vi "ATA_RT_2017_07_28.vi"() -> ()   [LabVIEW 2018]
doc: "This VI transfers a finite number of samples from the FPGA target to the Host using a stream."
uses:
  <vilib>/rvi/interface/nirviMethod/nirviMethod.xnode
  <vilib>/rvi/interface/nirviOpenFPGA/nirviOpenFPGA.xnode
  <vilib>/rvi/interface/nirviCloseFPGA/nirviCloseFPGA.xnode
  <vilib>/rvi/errors/niLvFpgaMergeErrorWithErrorCode.vi
  <vilib>/rvi/interface/nirviReadWriteControl/nirviReadWriteControl.xnode
  <vilib>/Analysis/NI_AALPro.lvlib
  <vilib>/FPGAPlugInAG/Dynamic/niLvFpga_ReadFifo_Dynamic.vi
  <vilib>/rvi/Analysis/host/Public/NI_FpgaMspHost.lvlib
  <vilib>/Analysis/2dsp.llb/Real FFT.vi
  <vilib>/FPGAPlugInAG/Dynamic/niLvFpga_StartFifo_Dynamic.vi
  <vilib>/rvi/interface/Simulation/niFpgaSimulationCallBeginRW.vi
  <vilib>/rvi/errors/niLvFpgaAdjustHostInterfaceError.vi
  ProjectFiles/FPGA Bitfiles/20170803_00_ATA_FPGA_00.lvbitx
  <vilib>/FPGAPlugInAG/Dynamic/niLvFpga_ConfigureFifo_Dynamic.vi
  NiFpgaLv.dll
  <vilib>/FPGAPlugInAG/Dynamic/niLvFpga_Close_Dynamic.vi
  Controls/DataClass.ctl
  <vilib>/Analysis/4window.llb/Hanning Window (DBL).vi
  Controls/ToneInfoClust.ctl
  <vilib>/FPGAPlugInAG/PXIe-7976R/niLvFpga_Open_PXIe-7976R.vi
  <vilib>/rvi/interface/common/dynamic/niFpgaDynamicAddResources.vi
panel:
  out "concatenated string":string
  out "FreqShiftTab":enum32{"Auto", "Manual"}(tab)=enum."Manual"
  in  "CoarseShift":dbl(slide)=-24999000.0 caption="Frequency Shift Coarse (Hz)" scale=-26000000.0..-23000000.0 scale format="%^#_6g"
  in  "FineShift":dbl(slide)=-462.63345195729516 caption="Frequency Shift Fine (Hz)" scale=-10000.0..10000.0 scale format="%^#_6g"
  in  "ProbesTab":T1(tab)=enum."Enable Stages"
  in  "EnableStep1":bool=TRUE
  in  "ScaleMeasurement":fxp<+/-,23,23>=10000.0
  in  "Scale_In_RT":ext=1.0
  in  "Scale_Step1":fxp<+/-,23,23>=4194303.0
  in  "Scale_NoiseFloor":fxp<+/-,23,23>=4194303.0
  in  "Offset":fxp<+/-,16,1>=0.000213623046875
  in  "FlushQ":bool=TRUE
  in  "Enable":T2={"FreqShiftEnable"=TRUE, "Step4Enable"=TRUE, "Step5Enable"=TRUE, "Step6Enable"=TRUE, "Step7Enable"=TRUE}
  in  "Scale":T3={"Scale_Step4"=10.0, "Scale_Step5"=1.0, "Scale_Step6"=1.0, "Scale_Step7"=1.0}
  out "Probe 1":i16=-13
  out "Probe 2":fxp<+/-,16,1>=-0.000274658203125
  out "Probe 3":fxp<+/-,39,24>=1.52587890625
  out "Probe 4":fxp<+/-,16,1>
  out "Probe 5":fxp<+/-,40,2>=-0.004281044006347656
  out "Probe 6":fxp<+/-,63,25>=9180.997811079025
  out "Probe 7":fxp<+/-,63,1>=6.103514169808477e-05
  out "Probe 21":fxp<+/-,24,3>=0.008556365966796875 format="%.2p"
  out "Probe 22":fxp<+/-,47,26>=4411.998948097229
  out "Probe 23":fxp<+/-,47,1>=-0.0003757475910788344
  out "Probe 24":fxp<+/-,16,1>=0.000213623046875
  out "Probe":T4={"Probe 8"=0.00049591064453125, "Probe 9"=0.0051984291058033705, "Probe 10"=0.051984291058033705, "Probe 11"=0.023252144874277292, "Probe 12"=0.023252144874277292, "Probe 13"=0.023252144874277292, "Probe 14"=0.015486729560507229, "Probe 15"=0.015486729560507229, "Probe 16"=0.015486729560507229, "Probe 17"=0.003276327208368457, "Probe 18"=0.003276327208368457, "Probe 19"=0.003276327208368457, "Probe20"=0.003276327208368457}
  out "TransferCount":u64=226407353343
  out "#Transfers":i32=74
  out "#FFTs":i32=74
  out "Elements Remaining":u32
  out "Peak Location":dbl=25000106.633451957 format="%^#_11g"
  out "SampleRate":dbl=12500.0
  out "max value":dbl=4.648353358875404e-06
  out "max index(es)":i32=644
  out "FAM Initialized?":bool=TRUE
  out "Total Shift":dbl=-24999462.633451957
  in  "AutoCenter":bool
  in  "Tab Control 2":T5(tab)
  out "NoiseFloor 2":ext[](graph)
  out "NoiseFloor":dbl[](graph)
  out "df (Hz) 2":dbl=7629.39453125
  out "NoiseFloorLoopCount":i32=77
  in  "Noise Floor":u8(slide)=1 scale=0.0..1.0
  out "TimeDomain":ext[](graph)
  out "Filtered Spectrum":dbl[](graph)
  out "df (Hz)":dbl=1.0
  in  "Zoom On Peak":bool
  in  "Tones":u8(slide)=1 scale=0.0..1.0
  in  "stop":bool
  # "Log"
  # "Linear"
  # "Log"
  # "Linear"
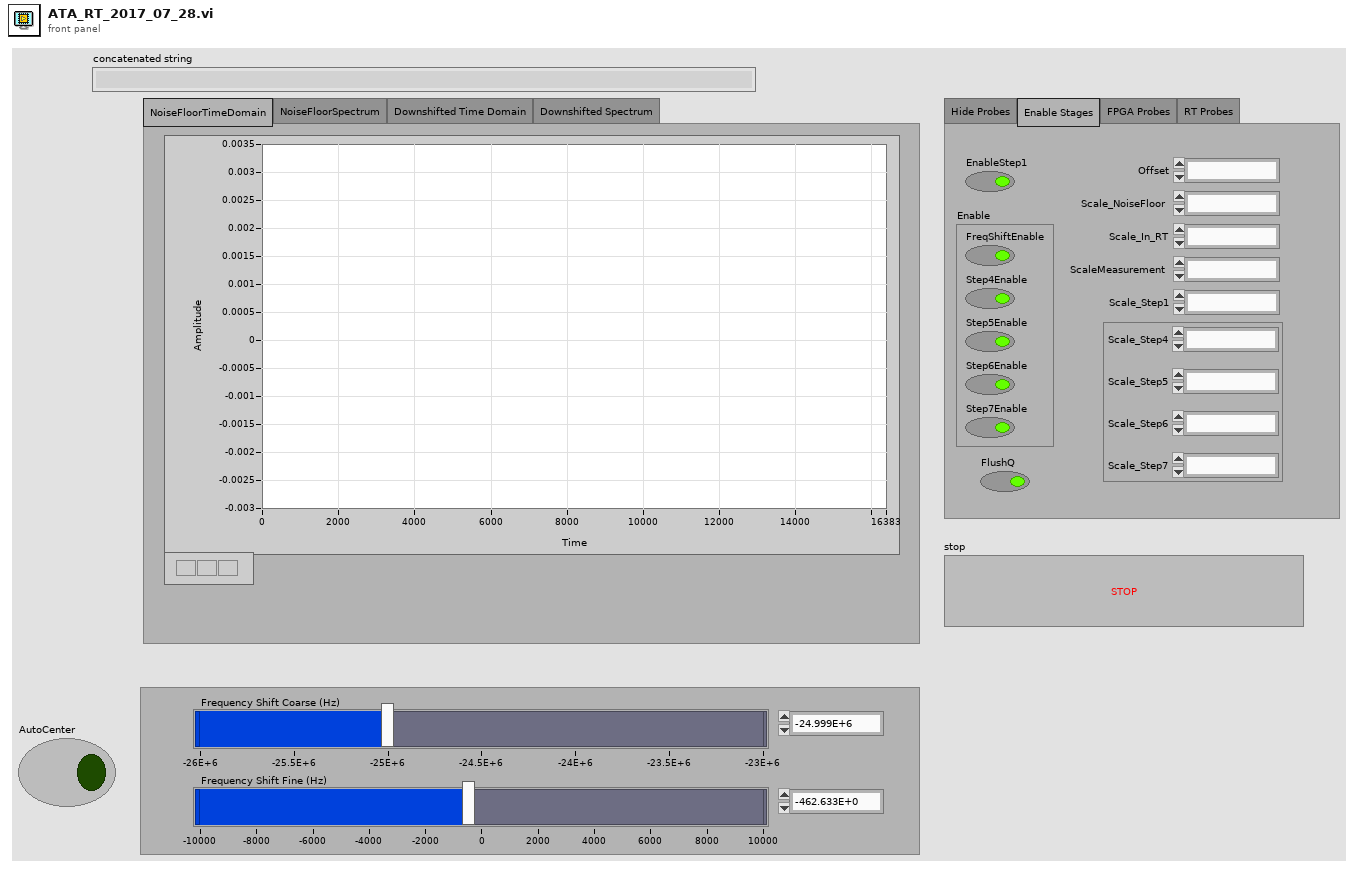
[diagram p1: front panel]
types:
  T1 = enum32{"Hide Probes", "Enable Stages", "FPGA Probes", "RT Probes"}
  T2 = cluster{"FreqShiftEnable":bool, "Step4Enable":bool, "Step5Enable":bool, "Step6Enable":bool, "Step7Enable":bool}
  T3 = cluster{"Scale_Step4":fxp<+/-,23,23>, "Scale_Step5":fxp<+/-,23,23>, "Scale_Step6":fxp<+/-,23,23>, "Scale_Step7":fxp<+/-,23,23>}
  T4 = cluster{"Probe 8":fxp<+/-,18,1>, "Probe 9":fxp<+/-,40,1>, "Probe 10":fxp<+/-,40,1>, "Probe 11":fxp<+/-,40,1>, "Probe 12":fxp<+/-,63,24>, "Probe 13":fxp<+/-,40,1>, "Probe 14":fxp<+/-,40,1>, "Probe 15":fxp<+/-,63,24>, "Probe 16":fxp<+/-,40,1>, "Probe 17":fxp<+/-,40,1>, "Probe 18":fxp<+/-,63,24>, "Probe 19":fxp<+/-,40,1>, "Probe20":fxp<+/-,40,1>}
  T5 = enum32{"NoiseFloorTimeDomain", "NoiseFloorSpectrum", "Downshifted Time Domain", "Downshifted Spectrum"}
  T6 = enum16{"open", "replace", "create", "open or create", "replace or create", "replace or create with confirmation"}
  T7 = typedef "DataClass.ctl" = enum16{"Tone", "Noise"}
  T8 = typedef "ToneInfoClust.ctl" = cluster{"PkLocTrak":dbl, "PkLocDisp":dbl, "df_":dbl, "ZoomPwr":dbl[], "Phase":dbl, "PhaseOld":dbl, "AboveThresh?":bool, "MaxI":dbl, "MaxQ":dbl, "median":dbl, "ISpect":dbl[], "QSpect":dbl[], "DeltaPhase":dbl}
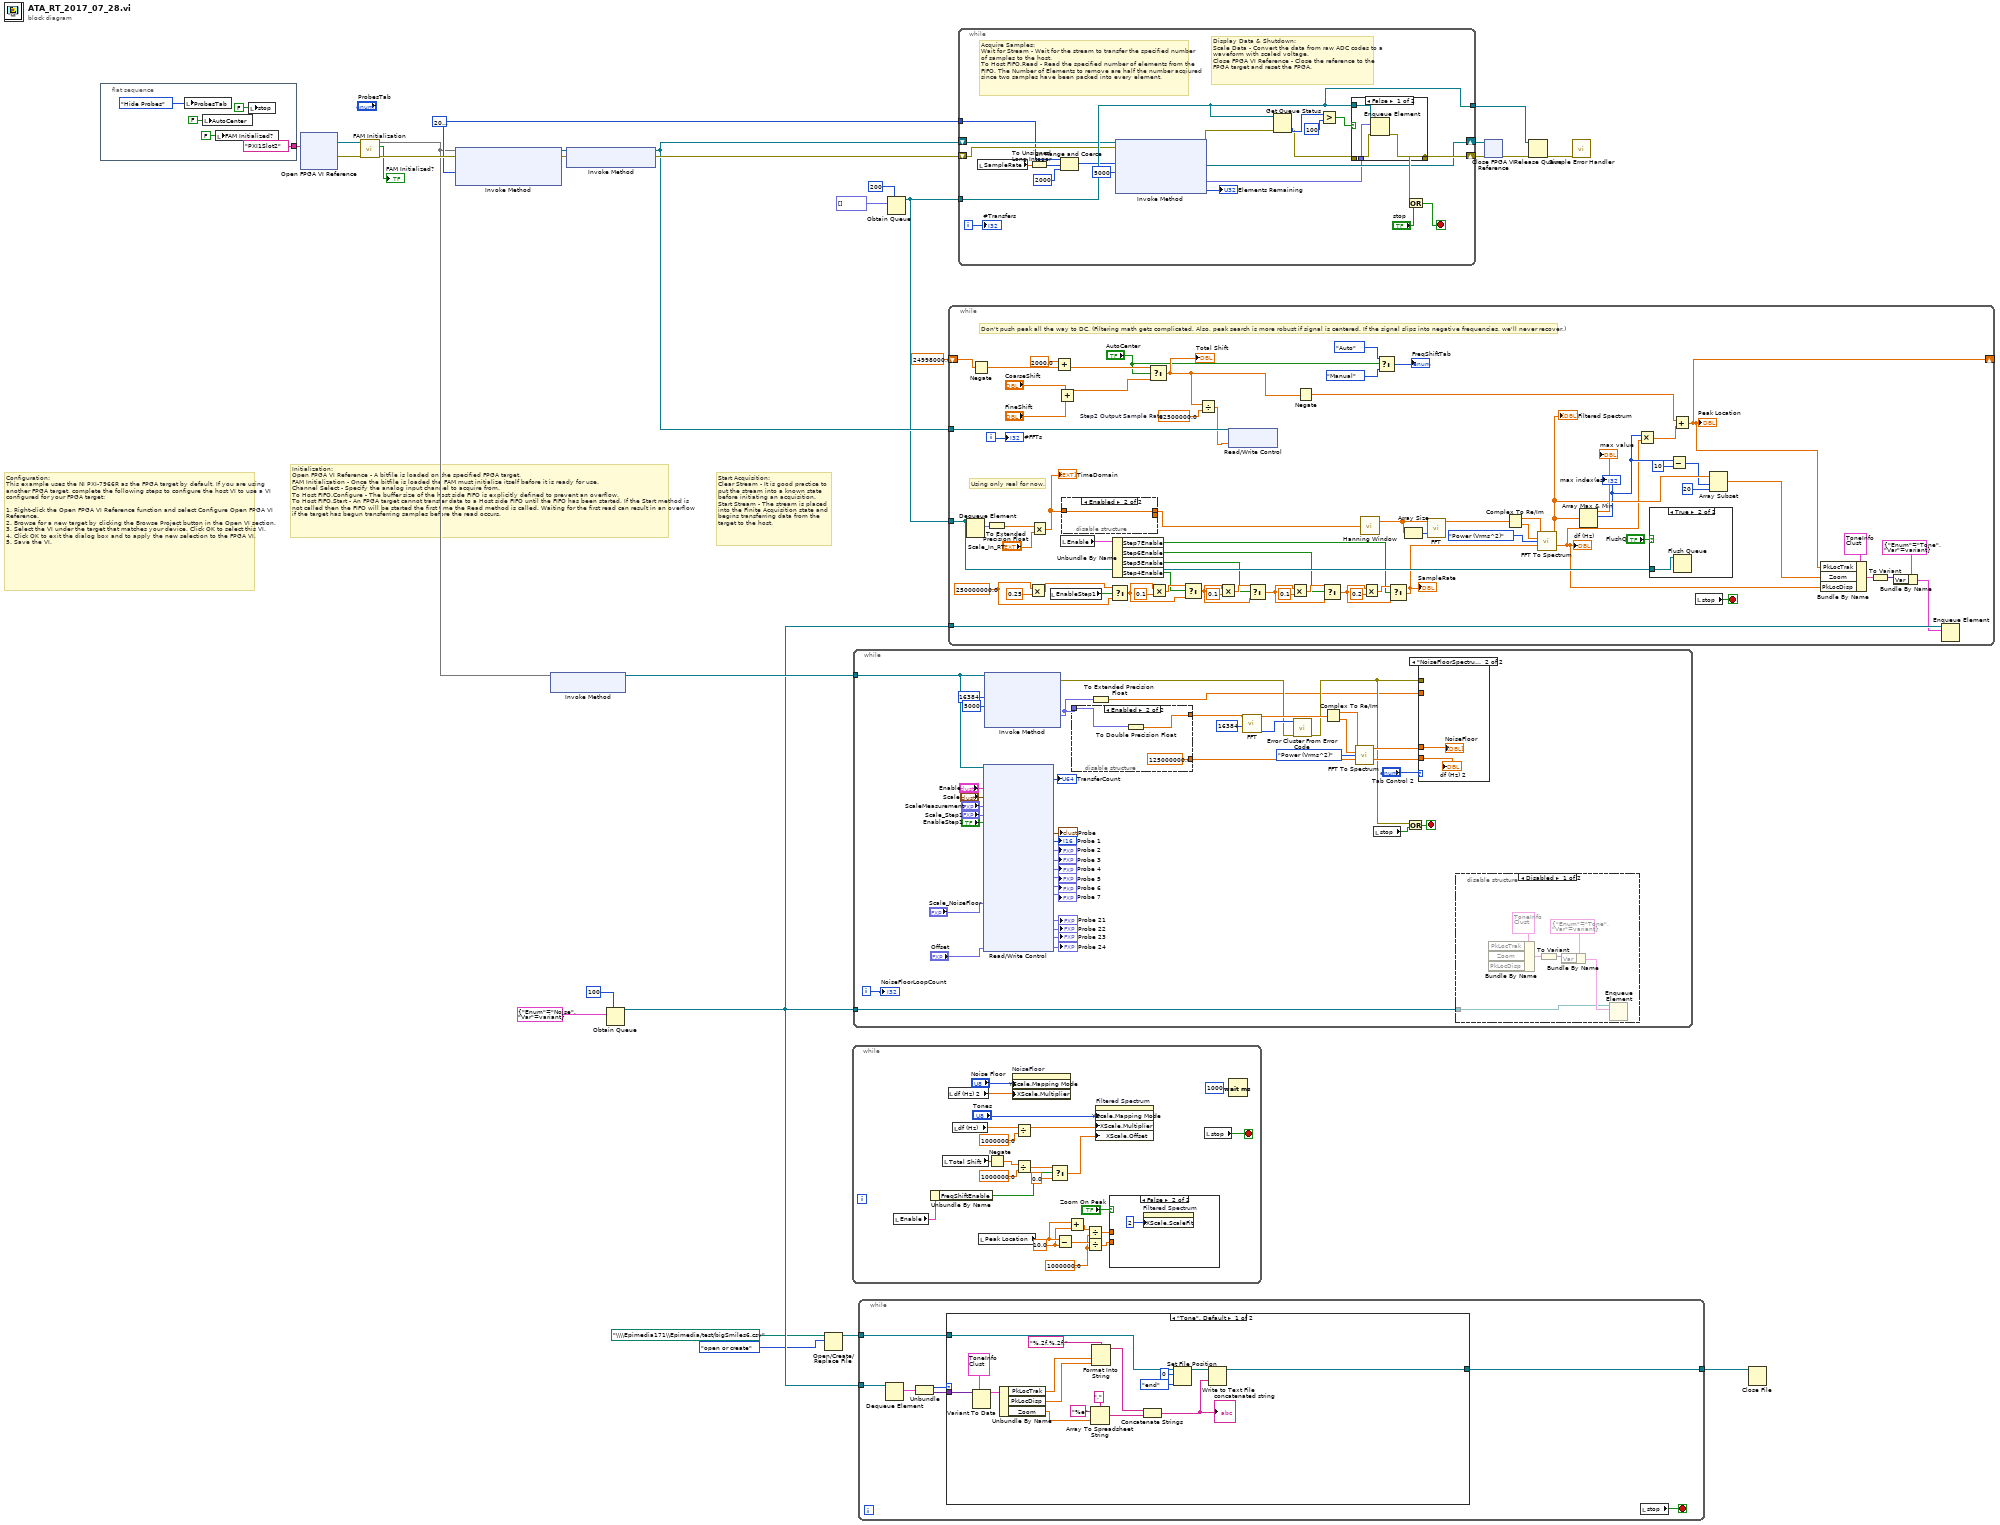
[diagram p0: block diagram]
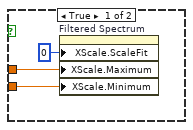
[diagram p3: hidden frame]
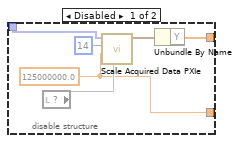
[diagram p5: hidden frame]
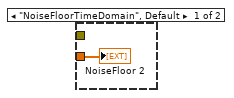
[diagram p6: hidden frame]
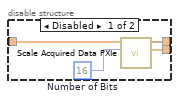
[diagram p7: hidden frame]
diagram:
  w18 = u32 2000000 ("Num Samples")
  # "Start Acquisition:\nClear Stream - It is good practice to put the stream into a known state before initiating an acquisition.\nStart Stream - The stream is placed into the Finite Acquisition state and begins transferring data from the target to the host."
  # "Initialization:\nOpen FPGA VI Reference - A bitfile is loaded on the specified FPGA target.\nFAM Initialization - Once the bitfile is loaded the FAM must initialize itself before it is ready for use.\nChannel Select - Specify the analog input channel to acquire from.\nTo Host FIFO.Configure - The buffer size of the host side FIFO is explicitly defined to prevent an overflow.\nTo Host FIFO.Start - An FPGA target cannot transfer data to a Host side FIFO until the FIFO has been started. If the Start method is not called then the FIFO will be started the first time the Read method is called. Waiting for the first read can result in an overflow if the target has begun transferring samples before the read occurs."
  # "Configuration:\nThis example uses the NI PXI-7966R as the FPGA target by default. If you are using another FPGA target, complete the following steps to configure the host VI to use a VI configured for your FPGA target:\n\n1. Right-click the Open FPGA VI Reference function and select Configure Open FPGA VI Reference.\n2. Browse for a new target by clicking the Browse Project button in the Open VI section.\n3. Select the VI under the target that matches your device. Click OK to select this VI.\n4. Click OK to exit the dialog box and to apply the new selection to the FPGA VI.\n5. Save the VI."
  n1 = flat-sequence {
    tunnel: [tag "PXI1Slot2" ("resource name")] -> w9
    frame #0 {
      n2 = local write "ProbesTab"(T1."Hide Probes" ("ProbesTab")) -> ()
      n3 = local write "AutoCenter"(FALSE ("AutoCenter")) -> ()
      n4 = local write "FAM Initialized?"(FALSE ("FAM Initialized?")) -> ()
      n5 = local write "stop"(FALSE ("stop")) -> ()
    }
  }
  n6 = xnode ("Open FPGA VI Reference")("resource name"=w9) -> ("FPGA VI Reference Out"=w19:refnum<k20>, "error out"=w24:errorcluster)  [unwired: 1 in]
  n7 = call "FAM Initialization.vi"("error in (no error)"=w24, "Cluster"=w19) -> ("error out"=w28:errorcluster, "FAM Initialized?"=→"FAM Initialized?":bool, 3:w11)  [unwired: 7 in]
  n8 = xnode "Invoke Method"("FPGA VI Reference In"=w11, "error in"=w28, "Requested Depth"=w18) -> ("FPGA VI Reference Out"=w26:refnum<k20>, "error out"=w25:errorcluster)  [unwired: 1 out]
  n9 = xnode "Invoke Method"("FPGA VI Reference In"=w11) -> ("FPGA VI Reference Out"=w10:refnum<k20>)  [unwired: 1 in, 1 out]
  n10 = xnode "Invoke Method"("FPGA VI Reference In"=w26, "error in"=w25) -> ("FPGA VI Reference Out"=w22:refnum<k20>, "error out"=w23:errorcluster)
  n11 = Obtain Queue(max queue size (-1, unlimited)=100, element data type=cluster{"Enum":T7, "Var":variant} {"Enum"=enum."Noise", "Var"=variant}) -> (queue out=w5:refnum<queue>)  [unwired: 3 in, 2 out]
  n12 = Open/Create/Replace File(file path (use dialog)=path "\\\\Epimedia171\\Epimedia/test/bigSmiles6.csv" ("file (use dialog)"), operation (0:open)=T6."open or create") -> (refnum out=w3:refnum<file>)  [unwired: 4 in, 2 out]
  n13 = while {
    stop <- w57 stop-if-true
    w39 = 1000000.0 ("x")
    w45 = 10.0 ("y")
    n14 = local read "Enable"() -> (w36:T2)
    n15 = Unbundle By Name(w36) -> ("FreqShiftEnable"=w35:bool)
    n16 = local read "Total Shift"() -> (w51:dbl)
    n17 = local read "df (Hz) 2"() -> (w52:dbl)
    n18 = local read "df (Hz)"() -> (w53:dbl)
    n19 = local read "Peak Location"() -> (w46:dbl)
    n20 = Negate(x=w51) -> (-x=w48:dbl)
    n21 = property on="NoiseFloor" class="WFGraph (strict)"("YScale.Mapping Mode"="Noise Floor", "XScale.Multiplier"=w52) -> ()  [unwired: 2 in, 2 out]
    n22 = Divide(x=w53, y=1000000.0) -> (x/y=w50:dbl)
    n23 = Divide(x=w48, y=1000000.0) -> (x/y=w38:dbl)
    n24 = Select(t=w38, s=w35, f=0.0) -> (s? t:f=w37:dbl)
    n25 = Subtract(x=w46, y=w45) -> (x-y=w41:dbl)
    n26 = Add(x=w46, y=w45) -> (x+y=w44:dbl)
    n27 = Divide(x=w44, y=w39) -> (x/y=w42:dbl)
    n28 = Divide(x=w41, y=w39) -> (x/y=w40:dbl)
    n29 = property on="Filtered Spectrum" class="WFGraph (strict)"("YScale.Mapping Mode"="Tones", "XScale.Multiplier"=w50, "XScale.Offset"=w37) -> ()  [unwired: 2 in, 2 out]
    n30 = case shown="False" "Zoom On Peak" {
      tunnel: w40 -> [w60 _]
      tunnel: w42 -> [w59 _]
      frame True {
        n31 = property on="Filtered Spectrum" class="WFGraph (strict)"("XScale.ScaleFit"=u8 0 ("X Scale.Scale Fit"), "XScale.Maximum"=w59, "XScale.Minimum"=w60) -> ()  [unwired: 2 in, 2 out]
      }
      frame False {
        n32 = property on="Filtered Spectrum" class="WFGraph (strict)"("XScale.ScaleFit"=u8 2 ("X Scale.Scale Fit")) -> ()  [unwired: 2 in, 2 out]
      }
    }
    n33 = local read "stop"() -> (w57:bool)
    n34 = Wait (ms)(milliseconds to wait=u32 1000) -> ()  [unwired: 1 out]
  }
  n35 = while {
    tunnel: w10 -> [w86]
    tunnel: w5 -> [w62]
    i -> [w92]
    stop <- w90 stop-if-true
    n36 = xnode "Read/Write Control"("FPGA VI Reference In"=w86, "Enable"="Enable", "Scale"="Scale", "ScaleMeasurement"="ScaleMeasurement", "Scale_Step1"="Scale_Step1", "EnableStep1"="EnableStep1", "Scale_NoiseFloor"="Scale_NoiseFloor", "Offset"="Offset") -> ("TransferCount"=→"TransferCount":u64, "Probe"=→"Probe":T4, "Probe 1"=→"Probe 1":i16, "Probe 2"=→"Probe 2":fxp<+/-,16,1>, "Probe 3"=→"Probe 3":fxp<+/-,39,24>, "Probe 4"=→"Probe 4":fxp<+/-,16,1>, "Probe 5"=→"Probe 5":fxp<+/-,40,2>, "Probe 6"=→"Probe 6":fxp<+/-,63,25>, "Probe 7"=→"Probe 7":fxp<+/-,63,1>, "Probe 21"=→"Probe 21":fxp<+/-,24,3>, "Probe 22"=→"Probe 22":fxp<+/-,47,26>, "Probe 23"=→"Probe 23":fxp<+/-,47,1>, "Probe 24"=→"Probe 24":fxp<+/-,16,1>)  [unwired: 1 in, 2 out]
    n37 = xnode "Invoke Method"("FPGA VI Reference In"=w86, "Number of Elements"=u32 16384, "Timeout (ms)"=5000) -> ("error out"=w88:errorcluster, "Data"=w84:fxp<+/-,16,1>[])  [unwired: 1 in, 2 out]
    n38 = disable-structure shown="Enabled" {
      disable-tunnel: [w115 w118] -> w94
      disable-tunnel: w84 -> [w114 w119]
      disable-tunnel: [w112 125000000.0 ("sample rate (S/s)")] -> w81
      frame Disabled {
        w112 = 125000000.0
        n39 = local read item#-1() -> (w116)
        n40 = call "Scale Acquired Data PXIe.vi"("range (V)"=w116, "Sample Rate"=w112, "Number of Bits"=i16 14, "Data In"=w114) -> ("Data Out"=w113:waveform(dbl))  [unwired: 6 in, 1 out]
        n41 = Unbundle By Name(w113) -> ("Y"=w115:dbl[])
      }
      frame Enabled {
        n42 = To Double Precision Float(number=w119) -> (double precision float=w118:dbl[])
      }
    }
    n43 = To Extended Precision Float(1:w84) -> (0:w83:ext[])
    n44 = call-poly <vilib>:"FFT.vi"("FFT size"=16384, "X"=w94) -> ("error"=w89:i32, "FFT {X}"=w98:cdb[])  [unwired: 8 in]
    n45 = call <vilib>:"Error Cluster From Error Code.vi"("error in (no error)"=w88, "error code (0)"=w89) -> ("error out"=w87:errorcluster)  [unwired: 7 in]
    n46 = Complex To Re/Im(x + iy=w98) -> (x=w99:dbl[], y=w100:dbl[])
    n47 = call <vilib>:"FFT To Spectrum.vi"("real FFT data"=w99, "imaginary FFT data"=w100, "spectrum type"=enum8{"Power (Vrms^2)", "Amplitude (Vrms)"}."Power (Vrms^2)", "sample rate (S/s)"=w81) -> ("spectrum out"=w97:dbl[], "df (Hz)"=w96:dbl)  [unwired: 9 in, 1 out]
    n48 = local read "stop"() -> (w91:bool)
    n49 = Or(x=w87, y=w91) -> (x .or. y?=w90:bool)
    n50 = case shown="\"NoiseFloorSpectrum\"" "Tab Control 2" {
      tunnel: w97 -> [_ w122]
      tunnel: w96 -> [_ w121]
      tunnel: w83 -> [w120 _]
      tunnel: w87 -> [_ _]
      frame "NoiseFloorTimeDomain", Default {
        "NoiseFloor 2" <- w120
      }
      frame "NoiseFloorSpectrum" {
        "NoiseFloor" <- w122
        "df (Hz) 2" <- w121
      }
    }
    n51 = disable-structure shown="Disabled" {
      disable-tunnel: w62 -> [w104 _]
      frame Disabled {
        n52 = Bundle By Name(cluster=T8 {"PkLocTrak"=0.0, "PkLocDisp"=0.0, "df_"=0.0, "ZoomPwr"=[], "Phase"=0.0, "PhaseOld"=0.0, "AboveThresh?"=FALSE, "MaxI"=0.0, "MaxQ"=0.0, "median"=0.0, "ISpect"=[], "QSpect"=[], "DeltaPhase"=0.0}) -> (w109:T8, "PkLocTrak"=w106:dbl)  [unwired: 2 in]
        n53 = To Variant(anything=w109) -> (Variant=w108:variant)
        n54 = Bundle By Name(cluster=cluster{"Enum":T7, "Var":variant} {"Enum"=enum."Tone", "Var"=variant} ("element"), "Var"=w108) -> (w110:cluster{"Enum":T7, "Var":variant})
        n55 = Enqueue Element(queue=w104, element=w110) -> ()  [unwired: 2 in, 3 out]
      }
      frame Enabled {
      }
    }
    "NoiseFloorLoopCount" <- w92
  }
  n56 = while {
    tunnel: w5 -> [w128]
    tunnel: w3 -> [w124]
    tunnel: [w123] -> w2
    stop <- w129 stop-if-true
    n57 = Dequeue Element(queue=w128) -> (element=w127:cluster{"Enum":T7, "Var":variant})  [unwired: 2 in, 3 out]
    n58 = Unbundle(w127) -> ("Enum"=w126:T7, "Var"=w125:variant)
    n59 = case shown="\"Tone\", Default" w126 {
      tunnel: w125 -> [w146 _]
      tunnel: w124 -> [w141 w147]
      tunnel: [w137 w147] -> w123
      frame "Tone", Default {
        n60 = Variant To Data(type=T8 {"PkLocTrak"=0.0, "PkLocDisp"=0.0, "df_"=0.0, "ZoomPwr"=[], "Phase"=0.0, "PhaseOld"=0.0, "AboveThresh?"=FALSE, "MaxI"=0.0, "MaxQ"=0.0, "median"=0.0, "ISpect"=[], "QSpect"=[], "DeltaPhase"=0.0}, Variant=w146) -> (data=w145:T8)  [unwired: 1 in, 1 out]
        n61 = Unbundle By Name(w145) -> ("PkLocTrak"=w133:dbl, "PkLocDisp"=w131:dbl, "Zoom"=w134:dbl[])
        n62 = Array To Spreadsheet String(delimiter (Tab)=",", array=w134, 3:"%e" ("format string")) -> (spreadsheet string=w136:string)
        n63 = Format Into String(format string="%.2f,%.2f,", w133, w131) -> (resulting string=w132:string)  [unwired: 2 in, 1 out]
        n64 = Concatenate Strings(w132, w136) -> (w135:string)
        "concatenated string" <- w135
        n65 = Set File Position(offset (in bytes) (0)=i64 0, refnum=w141, from (0:start)=enum16{"start", "end", "current"}."end") -> (refnum out=w140:refnum<file>)  [unwired: 1 in, 1 out]
        n66 = Write to Text File(file (use dialog)=w140, text=w135) -> (refnum out=w137:refnum<file>)  [unwired: 2 in, 2 out]
      }
      frame "Noise" {
      }
    }
    n67 = local read "stop"() -> (w129:bool)
  }
  n68 = Obtain Queue(max queue size (-1, unlimited)=200, element data type=fxp<+/-,40,3>[] [] ("Data")) -> (queue out=w15:refnum<queue>)  [unwired: 3 in, 2 out]
  n69 = while {
    tunnel: w15 -> [w215]
    tunnel: w22 -> [w212]
    shift-right: [w154] -> _
    shift-left: 24998000.0 -> [w177]
    tunnel: w5 -> [w156]
    i -> [w174]
    stop <- w216 stop-if-true
    w197 = 250000000.0 ("f")
    w200 = 62500000.0  # Step2 Output Sample Rate
    # "Don't push peak all the way to DC. (Filtering math gets complicated. Also, peak search is more robust if signal is centered. If the signal slips into negative frequencies, we'll never recover.)"
    # "Using only real for now."
    n70 = Dequeue Element(queue=w215) -> (element=w205:fxp<+/-,40,3>[])  [unwired: 2 in, 3 out]
    n71 = Negate(x=w177) -> (-x=w173:dbl)
    n72 = To Extended Precision Float(1:w205) -> (0:w203:ext[])
    n73 = Multiply(x=w197, y=0.25) -> (x*y=w198:dbl)
    n74 = Multiply(x=w203, y="Scale_In_RT") -> (x*y=w202:ext[])
    "TimeDomain" <- w202
    n75 = local read "EnableStep1"() -> (w182:bool)
    n76 = Add(x=2000.0, y=w173) -> (x+y=w176:dbl)
    n77 = Add(x="CoarseShift", y="FineShift") -> (x+y=w172:dbl)
    n78 = local read "Enable"() -> (w166:T2)
    n79 = disable-structure shown="Enabled" {
      disable-tunnel: [w217 w222] -> w207
      disable-tunnel: w202 -> [w218 w222]
      disable-tunnel: [w219 _] -> _
      frame Disabled {
        w221 = i16 16  # Number of Bits
        n80 = call "Scale Acquired Data PXIe.vi"("Number of Bits"=w221, "Data In"=w218) -> ("EXT_Values"=w219:ext[], "Data Out"=w217:waveform(dbl), "Sample Rate"=w220:dbl)  [unwired: 7 in]
      }
      frame Enabled {
      }
    }
    n81 = Select(t=w198, s=w182, f=w197) -> (s? t:f=w194:dbl)
    n82 = Unbundle By Name(w166) -> ("Step7Enable"=w162:bool, "Step6Enable"=w163:bool, "Step5Enable"=w164:bool, "Step4Enable"=w165:bool)
    n83 = Select(t=w176, s="AutoCenter", f=w172) -> (s? t:f=w171:dbl)
    "Total Shift" <- w171
    n84 = Multiply(x=w194, y=0.1) -> (x*y=w195:dbl)
    n85 = Select(t=w195, s=w165, f=w194) -> (s? t:f=w191:dbl)
    n86 = Divide(x=w171, y=w200) -> (x/y=w181:dbl)
    n87 = Multiply(x=w191, y=0.1) -> (x*y=w192:dbl)
    n88 = xnode "Read/Write Control"("FPGA VI Reference In"=w212, "FreqShiftCal"=w181) -> ()  [unwired: 1 in, 2 out]
    n89 = Select(t=w192, s=w164, f=w191) -> (s? t:f=w187:dbl)
    n90 = Multiply(x=w187, y=0.1) -> (x*y=w189:dbl)
    n91 = Negate(x=w171) -> (-x=w178:dbl)
    n92 = Select(t=w189, s=w163, f=w187) -> (s? t:f=w184:dbl)
    n93 = call-poly <vilib>:"Hanning Window.vi"("X"=w207) -> ("Windowed X"=w213:dbl[])  [unwired: 1 out]
    n94 = Multiply(x=w184, y=0.2) -> (x*y=w185:dbl)
    n95 = Select(t=enum32{"Auto", "Manual"}."Auto" ("FreqShiftTab"), s="AutoCenter", f=enum32{"Auto", "Manual"}."Manual" ("FreqShiftTab")) -> (s? t:f=→"FreqShiftTab":enum32{"Auto", "Manual"})
    n96 = Select(t=w185, s=w162, f=w184) -> (s? t:f=w183:dbl)
    "SampleRate" <- w183
    n97 = Array Size(array=w213) -> (size(s)=w206:i32)
    n98 = call-poly <vilib>:"FFT.vi"("FFT size"=w206, "X"=w213) -> ("FFT {X}"=w211:cdb[])  [unwired: 8 in, 1 out]
    n99 = Complex To Re/Im(x + iy=w211) -> (x=w210:dbl[], y=w209:dbl[])
    n100 = call <vilib>:"FFT To Spectrum.vi"("real FFT data"=w210, "imaginary FFT data"=w209, "spectrum type"=enum8{"Power (Vrms^2)", "Amplitude (Vrms)"}."Power (Vrms^2)", "sample rate (S/s)"=w183) -> ("spectrum out"=w161:dbl[], "df (Hz)"=w153:dbl)  [unwired: 9 in, 1 out]
    "df (Hz)" <- w153
    "Filtered Spectrum" <- w161
    n101 = Array Max & Min(array=w161) -> (max value=→"max value":dbl, max index (indices)=w160:i32)  [unwired: 2 out]
    "max index(es)" <- w160
    n102 = Multiply(x=w160, y=w153) -> (x*y=w179:dbl)
    n103 = case shown="True" "FlushQ" {
      tunnel: w215 -> [_ w223]
      frame False {
      }
      frame True {
        n104 = Flush Queue(queue=w223) -> ()  [unwired: 1 in, 3 out]
      }
    }
    n105 = Subtract(x=w160, y=10) -> (x-y=w158:i32)
    n106 = Add(x=w178, y=w179) -> (x+y=w154:dbl)
    "Peak Location" <- w154
    n107 = local read "stop"() -> (w216:bool)
    n108 = Array Subset(array=w161, index=w158, length=20) -> (w152:dbl[])
    n109 = Bundle By Name(cluster=T8 {"PkLocTrak"=0.0, "PkLocDisp"=0.0, "df_"=0.0, "ZoomPwr"=[], "Phase"=0.0, "PhaseOld"=0.0, "AboveThresh?"=FALSE, "MaxI"=0.0, "MaxQ"=0.0, "median"=0.0, "ISpect"=[], "QSpect"=[], "DeltaPhase"=0.0}, "PkLocTrak"=w154, "Zoom"=w152, "PkLocDisp"=w153) -> (w149:T8)
    n110 = To Variant(anything=w149) -> (Variant=w150:variant)
    n111 = Bundle By Name(cluster=cluster{"Enum":T7, "Var":variant} {"Enum"=enum."Tone", "Var"=variant} ("element"), "Var"=w150) -> (w148:cluster{"Enum":T7, "Var":variant})
    n112 = Enqueue Element(queue=w156, element=w148) -> ()  [unwired: 2 in, 3 out]
    "#FFTs" <- w174
  }
  n113 = while {
    tunnel: w18 -> [w228]
    shift-right: [w232] -> w21
    shift-left: w22 -> [w233]
    shift-right: [w236] -> w20
    shift-left: w23 -> [w230]
    tunnel: w15 -> [w234]
    tunnel: [w234] -> w13
    i -> [w242]
    stop <- w243 stop-if-true
    # "Display Data & Shutdown:\nScale Data - Convert the data from raw ADC codes to a waveform with scaled voltage.\nClose FPGA VI Reference - Close the reference to the FPGA target and reset the FPGA."
    # "Acquire Samples:\nWait for Stream - Wait for the stream to transfer the specified number of samples to the host.\nTo Host FIFO.Read - Read the specified number of elements from the FIFO. The Number of Elements to remove are half the number acqiured since two samples have been packed into every element."
    n114 = local read "SampleRate"() -> (w227:dbl)
    n115 = To Unsigned Long Integer(number=w227) -> (unsigned 32bit integer=w224:u32)
    n116 = In Range and Coerce(upper limit=w228, x=w224, lower limit=u32 2000) -> (coerced(x)=w226:u32)  [unwired: 1 out]
    n117 = xnode "Invoke Method"("FPGA VI Reference In"=w233, "error in"=w230, "Number of Elements"=w226, "Timeout (ms)"=5000) -> ("FPGA VI Reference Out"=w232:refnum<k20>, "error out"=w238:errorcluster, "Data"=w229:fxp<+/-,40,1>[], "Elements Remaining"=→"Elements Remaining":u32)
    n118 = Get Queue Status(queue=w234, error in (no error)=w238) -> (error out=w237:errorcluster, # elements in queue=w240:i32)  [unwired: 1 in, 6 out]
    n119 = Greater?(x=w240, y=100) -> (0:w235:bool)
    n120 = case shown="False" w235 {
      tunnel: w229 -> [w248 _]
      tunnel: w234 -> [w247 _]
      tunnel: w237 -> [w246 w249]
      tunnel: [w245 w249] -> w236
      frame False {
        n121 = Enqueue Element(queue=w247, element=w248, error in (no error)=w246) -> (error out=w245:errorcluster)  [unwired: 1 in, 2 out]
      }
      frame True {
      }
    }
    n122 = Or(x=w236, y="stop") -> (x .or. y?=w243:bool)
    "#Transfers" <- w242
  }
  n123 = xnode ("Close FPGA VI Reference")("FPGA VI Reference In"=w21, "error in"=w20) -> ("error out"=w17:errorcluster)
  n124 = Release Queue(queue=w13, error in (no error)=w17) -> (error out=w16:errorcluster)  [unwired: 1 in, 2 out]
  n125 = call <vilib>:"Simple Error Handler.vi"("error in (no error)"=w16) -> ()  [unwired: 4 in, 5 out]
  n126 = Close File(refnum=w2) -> ()  [unwired: 1 in, 2 out]
